vi "Test_OpenConnectionBadCredentials_ReturnsError.vi"(8 "error in (no error)":errorcluster, 11 "TestCase in":refnum<class "Test mysql.lvclass">) -> (0 "error out":errorcluster, 3 "TestCase out":refnum<class "Test mysql.lvclass">)   [LabVIEW 2020, in "DataBase_mysql_Tests.lvlib" / "Test mysql.lvclass"]
uses:
  Test mysql.lvclass
  externals/mysql/Source/mysql.net/mysql.lvclass
  <vilib>/addons/_JKI Toolkits/VI Tester/TestCase.llb/TestCase.lvclass
  C:/Program Files/National Instruments/LabVIEW 2020/vi.lib/addons/_JKI Toolkits/VI Tester/TestCase.llb/TestCase.lvclass
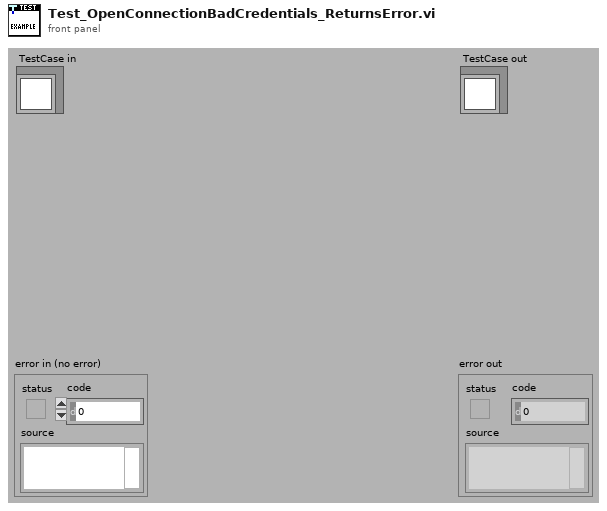
[diagram p1: front panel]
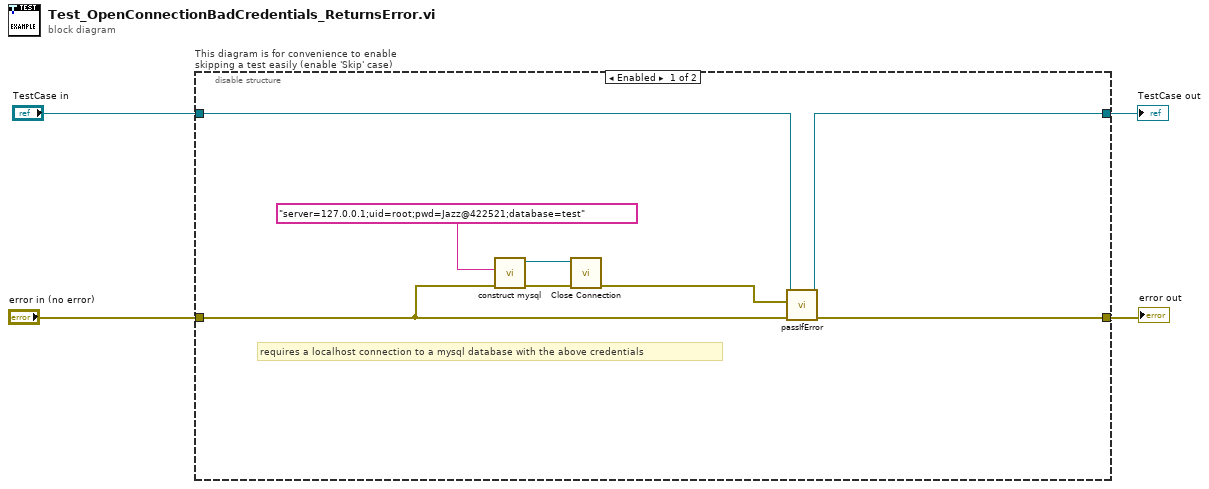
[diagram p0: block diagram]
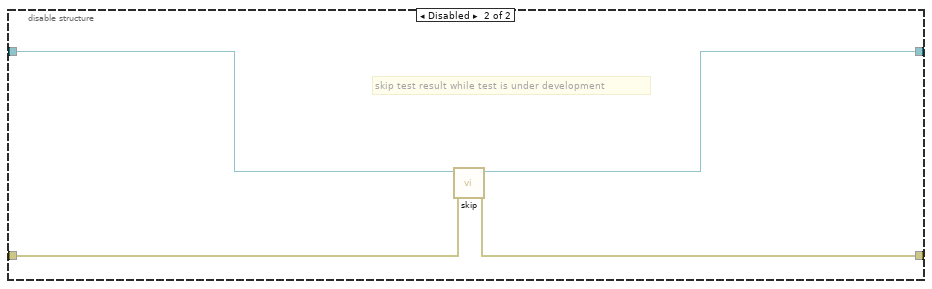
[diagram p2: hidden frame]
diagram:
  n1 = disable-structure "This diagram is for convenience to enable skipping a test easily (enable 'Skip' case)" shown="Enabled" {
    disable-tunnel: "TestCase in" -> [w12 w16]
    disable-tunnel: [w11 w14] -> w1
    disable-tunnel: [w10 w15] -> w3
    disable-tunnel: "error in (no error)" -> [w6 w13]
    frame Enabled {
      # "requires a localhost connection to a mysql database with the above credentials"
      n2 = call "construct mysql.vi"("error in (no error)"=w6, "Connection string"="server=127.0.0.1;uid=root;pwd=Jazz@422521;database=test") -> ("error out"=w8:errorcluster, "mysql out"=w9:refnum<class "mysql.lvclass">)  [unwired: 8 in]
      n3 = call-dynamic "Close Connection.vi"("error in (no error)"=w8, "mysql in"=w9) -> ("error out"=w5:errorcluster)  [unwired: 8 in, 1 out]
      n4 = call-dynamic "passIfError.vi"("error in (no error)"=w6, "error"=w5, "TestCase in"=w12) -> ("error out"=w10:errorcluster, "TestCase out"=w11:refnum<class "Test mysql.lvclass">)  [unwired: 7 in]
    }
    frame Disabled {
      # "skip test result while test is under development"
      n5 = call <vilib>:"skip.vi"("error in (no error)"=w13, "TestCase in"=w16) -> ("error out"=w15:errorcluster, "TestCase out"=w14:refnum<class "Test mysql.lvclass">)  [unwired: 8 in]
    }
  }
  "error out" <- w3
  "TestCase out" <- w1
